vi "Telemetry Plotting test code.vi"() -> ()   [LabVIEW 2017]
panel:
  out "New Data":bool
  out "Plotting?":bool
  in  "PC To Rio":T1
  in  "XY Complete?":bool
  in  "stop":bool
  out "X Speed PID":cluster{"Speed SP":dbl, "Speed PV":dbl}(graph)
  out "Y Speed PID":cluster{"Speed SP":dbl, "Speed PV":dbl}(graph)
  out "XY Complete?":bool
  # "Works when commands changed, then reset XY complete immediately\nOtherwise stuck in plotting loop"
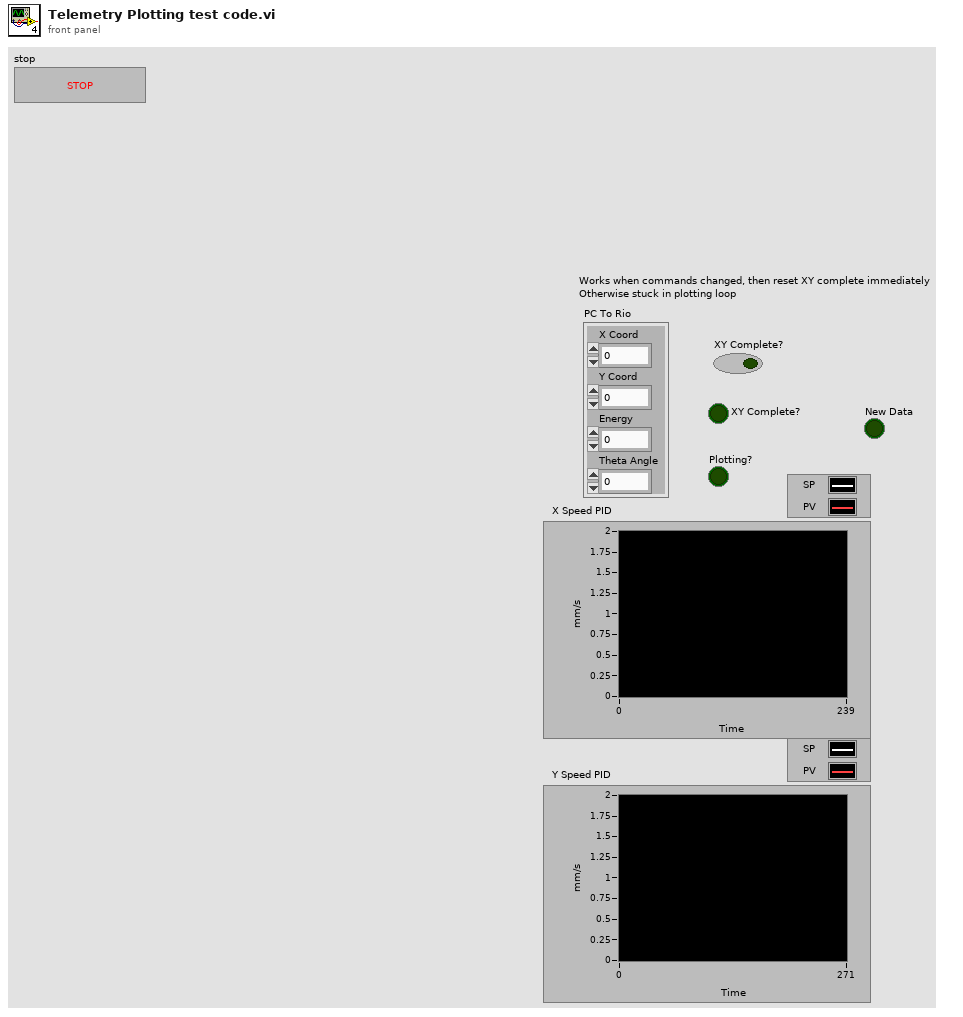
[diagram p1: front panel]
types:
  T1 = cluster{"X Coord":dbl, "Y Coord":dbl, "Energy":dbl, "Theta Angle":dbl}
  T2 = cluster{"X Coord":bool, "Y Coord":bool, "Energy":bool, "Theta Angle":bool}
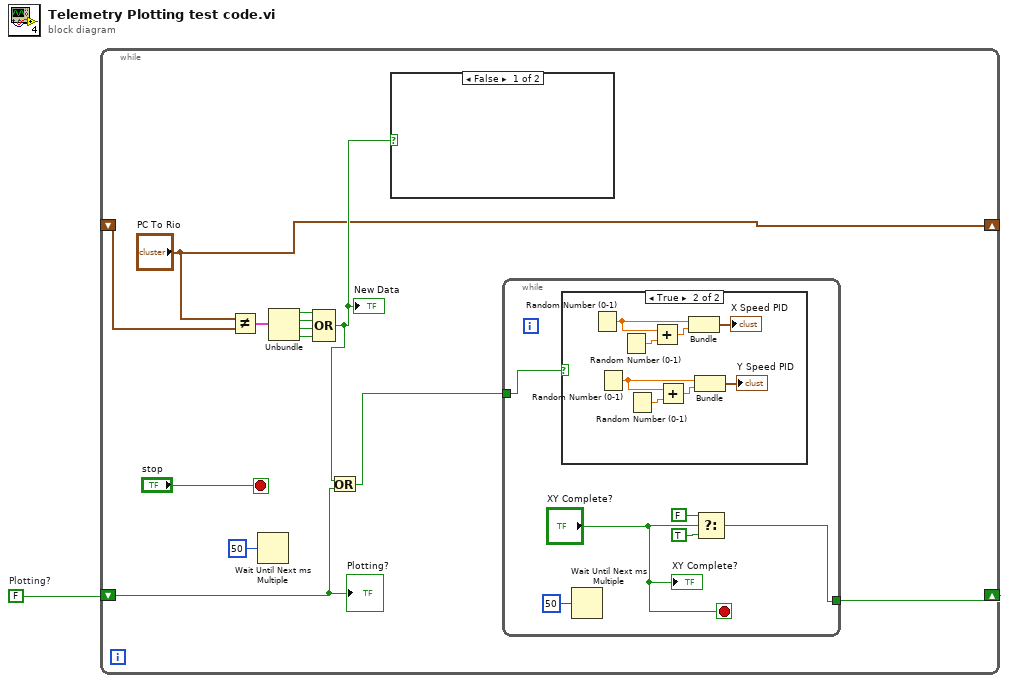
[diagram p0: block diagram]
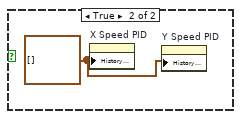
[diagram p3: hidden frame]
diagram:
  w1 = FALSE  # Plotting?
  n1 = while {
    shift-right: ["PC To Rio"] -> _
    shift-left: _ -> [w13]
    shift-right: [w4] -> _
    shift-left: w1 -> [w6]
    stop <- "stop" stop-if-true
    n2 = Not Equal?(x="PC To Rio", y=w13) -> (x != y?=w12:T2)
    n3 = Wait Until Next ms Multiple(millisecond multiple=u32 50) -> ()  [unwired: 1 out]
    n4 = Unbundle(w12) -> ("X Coord"=w11:bool, "Y Coord"=w10:bool, "Energy"=w9:bool, "Theta Angle"=w8:bool)
    n5 = Compound Arithmetic op=OR(w11, w10, w9, w8) -> (w7:bool)
    "New Data" <- w7
    n6 = Or(x=w7, y=w6) -> (x .or. y?=w3:bool)
    n7 = case shown="False" w7 {
      frame False {
      }
      frame True {
        w29 = cluster{"Speed SP":dbl, "Speed PV":dbl}[] [] ("History Data")
        n8 = property on="X Speed PID" class="WFChart (strict)"("History Data"=w29) -> ()  [unwired: 2 in, 2 out]
        n9 = property on="Y Speed PID" class="WFChart (strict)"("History Data"=w29) -> ()  [unwired: 2 in, 2 out]
      }
    }
    n10 = while {
      tunnel: [w17] -> w4
      tunnel: w3 -> [w16]
      stop <- "XY Complete?" stop-if-true
      n11 = case shown="True" w16 {
        frame False {
        }
        frame True {
          n12 = Random Number (0-1)() -> (number: 0 to 1=w28:dbl)
          n13 = Random Number (0-1)() -> (number: 0 to 1=w24:dbl)
          n14 = Random Number (0-1)() -> (number: 0 to 1=w27:dbl)
          n15 = Random Number (0-1)() -> (number: 0 to 1=w25:dbl)
          n16 = Add(x=w28, y=w27) -> (x+y=w26:dbl)
          n17 = Add(x=w24, y=w25) -> (x+y=w23:dbl)
          n18 = Bundle("number: 0 to 1"=w28, w26) -> (→"X Speed PID":cluster{"number: 0 to 1":dbl, dbl})  [unwired: 1 in]
          n19 = Bundle("number: 0 to 1"=w24, w23) -> (→"Y Speed PID":cluster{"number: 0 to 1":dbl, dbl})  [unwired: 1 in]
        }
      }
      n20 = Wait Until Next ms Multiple(millisecond multiple=u32 50) -> ()  [unwired: 1 out]
      n21 = Select(t=FALSE, s="XY Complete?", f=TRUE) -> (s? t:f=w17:bool)
      "XY Complete?" <- "XY Complete?"
    }
    "Plotting?" <- w6
  }
